vi "Rotate Boat Overlays.vi"(3 "Overlay References In":T1, 4 "SailPosition":dbl, 5 "Heading":dbl) -> (1 "Rotated Boat Icon Bitmap Out":u32[][](array[colorbox]), 2 "Boat Icon Out":T2(plugin-control))   [LabVIEW 2013]
doc: "Rotates icon images of the boat and sails and overlays them on each other to create a representation of the current state of the robot. Also converts the output image to a bitmap for easy overlay on the mission map.\n\norigininally by Jason Curtis\nAdapted 4/5/2014 by Mac-I Crowell"
uses:
  TypeDef/Overlay References.ctl
  <vilib>/vision/Image Controls.llb/IMAQ Image.ctl
  <vilib>/vision/NI_Vision_Development_Module.lvlib
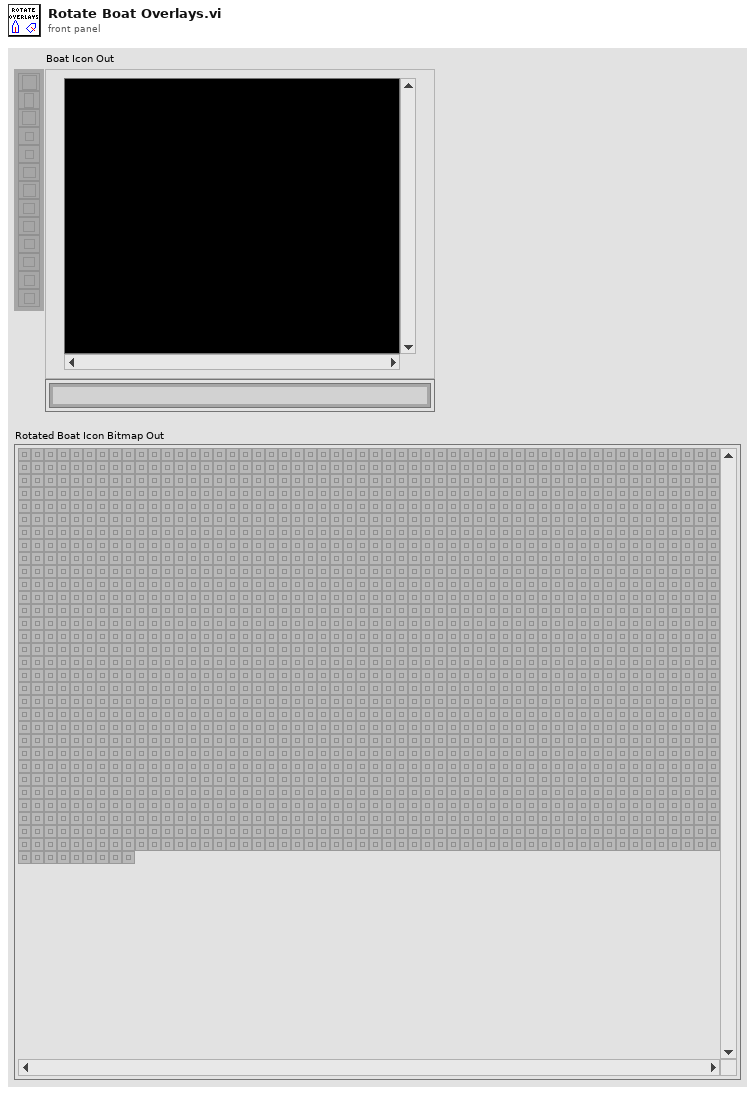
[diagram p1: front panel]
types:
  T1 = typedef "Overlay References.ctl" = cluster{"Boat Icon, Unroatated":T2, "Boat Icon, Rotated":T2, "Sail Icon, Unrotated":T2, "Sail Icon, Rotated":T2}
  T2 = typedef "IMAQ Image.ctl" = refnum<image>
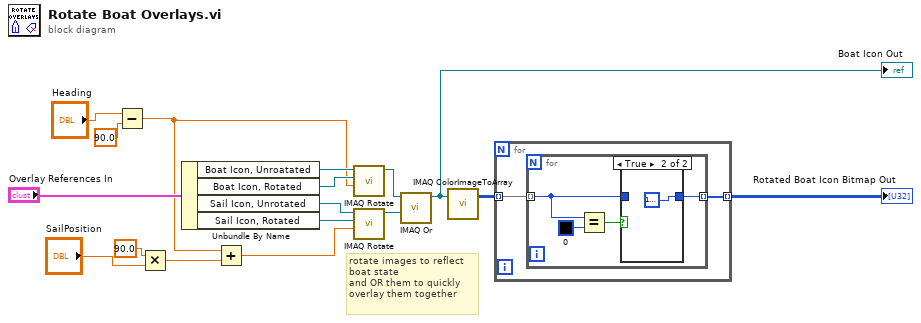
[diagram p0: block diagram]
diagram:
  # "rotate images to reflect\nboat state\nand OR them to quickly \noverlay them together"
  n1 = Subtract(x="Heading", y=90.0) -> (x-y=w4:dbl)
  n2 = Multiply(x=90.0 ("y"), y="SailPosition") -> (x*y=w6:dbl)
  n3 = Unbundle By Name("Overlay References In") -> ("Boat Icon, Unroatated"=w17:T2, "Boat Icon, Rotated"=w16:T2, "Sail Icon, Unrotated"=w14:T2, "Sail Icon, Rotated"=w15:T2)
  n4 = Add(x=w4, y=w6) -> (x+y=w7:dbl)
  n5 = call "IMAQ Rotate"("Angle (degrees)"=w4, "Image Dst"=w16, "Image Src"=w17) -> ("Image Dst Out"=w10:T2)  [unwired: 7 in, 1 out]
  n6 = call "IMAQ Rotate"("Angle (degrees)"=w7, "Image Dst"=w15, "Image Src"=w14) -> ("Image Dst Out"=w11:T2)  [unwired: 7 in, 1 out]
  n7 = call "IMAQ Or"("Image Src B"=w11, "Image Src A"=w10) -> ("Image Dst Out"=w12:T2)  [unwired: 8 in, 1 out]
  "Boat Icon Out" <- w12
  n8 = call "IMAQ ColorImageToArray"("Image"=w12) -> ("Image Pixels (U32)"=w8:u32[][])  [unwired: 2 in, 3 out]
  n9 = for {
    tunnel: w8 -> [w19] mode=indexing
    tunnel: [w18] -> w9 mode=indexing
    n10 = for {
      tunnel: w19 -> [w21] mode=indexing
      tunnel: [w22] -> w18 mode=indexing
      n11 = Equal?(x=w21, y=u32 0) -> (x = y?=w23:bool)
      n12 = case shown="True" w23 {
        tunnel: [w24 u32 16777216] -> w22
        tunnel: w21 -> [w24 _]
        frame False {
        }
        frame True {
        }
      }
    }
  }
  "Rotated Boat Icon Bitmap Out" <- w9
